vi "Diode-Open.vi"(8 "error in (no error)":errorcluster, 11 "IP Address of Diode":string="192.168.203.151") -> (0 "error out":errorcluster, 3 "connection ID":refnum<k5>)   [LabVIEW 2020]
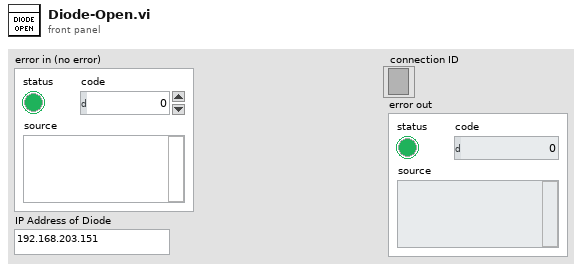
[diagram p1: front panel]
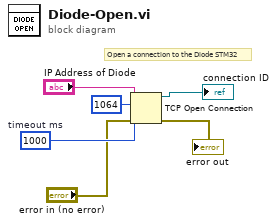
[diagram p0: block diagram]
diagram:
  w2 = 1000  # timeout ms
  # "Open a connection to the Diode STM32"
  n1 = TCP Open Connection(address="IP Address of Diode", remote port or service name=u16 1064, timeout ms (60000)=w2, error in (no error)="error in (no error)") -> (connection ID=→"connection ID":refnum<k5>, error out=→"error out":errorcluster)  [unwired: 1 in]
